vi "数字量输入配置.vi"() -> ()   [LabVIEW 2010]
uses:
  全局量/全局_配置.vi
panel:
  in  "数组":u16[](array[numeric]) format="%x"
  in  "保持输入":bool
  out "同步_A2":i32
  out "同步_A1":i32
  in  "数组_输入值":enum16{"0", "1"}[][](array[ring])
  in  "数组_选择?":bool[][](array[boolean])
  in  "btn_置1_5":bool
  in  "btn_置1_4":bool
  in  "btn_置1_3":bool
  in  "btn_置1_2":bool
  in  "btn_全选_5":bool
  in  "btn_全选_4":bool
  in  "btn_全选_3":bool
  in  "btn_全选_2":bool
  in  "btn_置1_1":bool
  in  "btn_全选_1":bool
  in  "CAN端口":u16
  out "light_80":bool
  out "light_79":bool
  out "light_78":bool
  out "light_77":bool
  out "light_76":bool
  out "light_75":bool
  out "light_74":bool
  out "light_73":bool
  out "light_72":bool
  out "light_71":bool
  out "light_70":bool
  out "light_69":bool
  out "light_68":bool
  out "light_67":bool
  out "light_66":bool
  out "light_65":bool
  in  "输入值_73":enum16{"0", "1"}(ring)
  in  "输入值_80":enum16{"0", "1"}(ring)
  in  "输入值_79":enum16{"0", "1"}(ring)
  in  "输入值_78":enum16{"0", "1"}(ring)
  in  "输入值_77":enum16{"0", "1"}(ring)
  in  "输入值_76":enum16{"0", "1"}(ring)
  in  "输入值_75":enum16{"0", "1"}(ring)
  in  "输入值_74":enum16{"0", "1"}(ring)
  in  "输入值_65":enum16{"0", "1"}(ring)
  in  "输入值_72":enum16{"0", "1"}(ring)
  in  "输入值_71":enum16{"0", "1"}(ring)
  in  "输入值_70":enum16{"0", "1"}(ring)
  in  "输入值_69":enum16{"0", "1"}(ring)
  in  "输入值_68":enum16{"0", "1"}(ring)
  in  "输入值_67":enum16{"0", "1"}(ring)
  in  "输入值_66":enum16{"0", "1"}(ring)
  in  "单选_第73路":bool
  in  "单选_第80路":bool
  in  "单选_第79路":bool
  in  "单选_第78路":bool
  in  "单选_第77路":bool
  in  "单选_第76路":bool
  in  "单选_第75路":bool
  in  "单选_第74路":bool
  in  "单选_第65路":bool
  in  "单选_第72路":bool
  in  "单选_第71路":bool
  in  "单选_第70路":bool
  in  "单选_第69路":bool
  in  "单选_第68路":bool
  in  "单选_第67路":bool
  in  "单选_第66路":bool
  out "light_64":bool
  out "light_63":bool
  out "light_62":bool
  out "light_61":bool
  out "light_60":bool
  out "light_59":bool
  out "light_58":bool
  out "light_57":bool
  out "light_56":bool
  out "light_55":bool
  out "light_54":bool
  out "light_53":bool
  out "light_52":bool
  out "light_51":bool
  out "light_50":bool
  out "light_49":bool
  in  "输入值_57":enum16{"0", "1"}(ring)
  in  "输入值_64":enum16{"0", "1"}(ring)
  in  "输入值_63":enum16{"0", "1"}(ring)
  in  "输入值_62":enum16{"0", "1"}(ring)
  in  "输入值_61":enum16{"0", "1"}(ring)
  in  "输入值_60":enum16{"0", "1"}(ring)
  in  "输入值_59":enum16{"0", "1"}(ring)
  in  "输入值_58":enum16{"0", "1"}(ring)
  in  "输入值_49":enum16{"0", "1"}(ring)
  in  "输入值_56":enum16{"0", "1"}(ring)
  in  "输入值_55":enum16{"0", "1"}(ring)
  in  "输入值_54":enum16{"0", "1"}(ring)
  in  "输入值_53":enum16{"0", "1"}(ring)
  in  "输入值_52":enum16{"0", "1"}(ring)
  in  "输入值_51":enum16{"0", "1"}(ring)
  in  "输入值_50":enum16{"0", "1"}(ring)
  in  "单选_第57路":bool
  in  "单选_第64路":bool
  in  "单选_第63路":bool
  in  "单选_第62路":bool
  in  "单选_第61路":bool
  in  "单选_第60路":bool
  in  "单选_第59路":bool
  in  "单选_第58路":bool
  in  "单选_第49路":bool
  in  "单选_第56路":bool
  in  "单选_第55路":bool
  in  "单选_第54路":bool
  in  "单选_第53路":bool
  in  "单选_第52路":bool
  in  "单选_第51路":bool
  in  "单选_第50路":bool
  out "light_48":bool
  out "light_47":bool
  out "light_46":bool
  out "light_45":bool
  out "light_44":bool
  out "light_43":bool
  out "light_42":bool
  out "light_41":bool
  out "light_40":bool
  out "light_39":bool
  out "light_38":bool
  out "light_37":bool
  out "light_36":bool
  out "light_35":bool
  out "light_34":bool
  out "light_33":bool
  in  "输入值_41":enum16{"0", "1"}(ring)
  in  "输入值_48":enum16{"0", "1"}(ring)
  in  "输入值_47":enum16{"0", "1"}(ring)
  in  "输入值_46":enum16{"0", "1"}(ring)
  in  "输入值_45":enum16{"0", "1"}(ring)
  in  "输入值_44":enum16{"0", "1"}(ring)
  in  "输入值_43":enum16{"0", "1"}(ring)
  in  "输入值_42":enum16{"0", "1"}(ring)
  in  "输入值_33":enum16{"0", "1"}(ring)
  in  "输入值_40":enum16{"0", "1"}(ring)
  in  "输入值_39":enum16{"0", "1"}(ring)
  in  "输入值_38":enum16{"0", "1"}(ring)
  in  "输入值_37":enum16{"0", "1"}(ring)
  in  "输入值_36":enum16{"0", "1"}(ring)
  in  "输入值_35":enum16{"0", "1"}(ring)
  in  "输入值_34":enum16{"0", "1"}(ring)
  in  "单选_第41路":bool
  in  "单选_第48路":bool
  in  "单选_第47路":bool
  in  "单选_第46路":bool
  in  "单选_第45路":bool
  in  "单选_第44路":bool
  in  "单选_第43路":bool
  in  "单选_第42路":bool
  in  "单选_第33路":bool
  in  "单选_第40路":bool
  in  "单选_第39路":bool
  in  "单选_第38路":bool
  in  "单选_第37路":bool
  in  "单选_第36路":bool
  in  "单选_第35路":bool
  in  "单选_第34路":bool
  out "light_32":bool
  out "light_31":bool
  out "light_30":bool
  out "light_29":bool
  out "light_28":bool
  out "light_27":bool
  out "light_26":bool
  out "light_25":bool
  out "light_24":bool
  out "light_23":bool
  out "light_22":bool
  out "light_21":bool
  out "light_20":bool
  out "light_19":bool
  out "light_18":bool
  out "light_17":bool
  in  "输入值_25":enum16{"0", "1"}(ring)
  in  "输入值_32":enum16{"0", "1"}(ring)
  in  "输入值_31":enum16{"0", "1"}(ring)
  in  "输入值_30":enum16{"0", "1"}(ring)
  in  "输入值_29":enum16{"0", "1"}(ring)
  in  "输入值_28":enum16{"0", "1"}(ring)
  in  "输入值_27":enum16{"0", "1"}(ring)
  in  "输入值_26":enum16{"0", "1"}(ring)
  in  "输入值_17":enum16{"0", "1"}(ring)
  in  "输入值_24":enum16{"0", "1"}(ring)
  in  "输入值_23":enum16{"0", "1"}(ring)
  in  "输入值_22":enum16{"0", "1"}(ring)
  in  "输入值_21":enum16{"0", "1"}(ring)
  in  "输入值_20":enum16{"0", "1"}(ring)
  in  "输入值_19":enum16{"0", "1"}(ring)
  in  "输入值_18":enum16{"0", "1"}(ring)
  in  "单选_第25路":bool
  in  "单选_第32路":bool
  in  "单选_第31路":bool
  in  "单选_第30路":bool
  in  "单选_第29路":bool
  in  "单选_第28路":bool
  in  "单选_第27路":bool
  in  "单选_第26路":bool
  in  "单选_第17路":bool
  in  "单选_第24路":bool
  in  "单选_第23路":bool
  in  "单选_第22路":bool
  in  "单选_第21路":bool
  in  "单选_第20路":bool
  in  "单选_第19路":bool
  in  "单选_第18路":bool
  in  "D_IN_5":string[][](table) caption="表格"
  in  "D_IN_4":string[][](table) caption="表格"
  in  "D_IN_3":string[][](table) caption="表格"
  in  "D_IN_2":string[][](table) caption="表格"
  out "light_16":bool
  out "light_15":bool
  out "light_14":bool
  out "light_13":bool
  out "light_12":bool
  out "light_11":bool
  out "light_10":bool
  out "light_9":bool
  out "light_8":bool
  out "light_7":bool
  out "light_6":bool
  out "light_5":bool
  out "light_4":bool
  out "light_3":bool
  out "light_2":bool
  out "light_1":bool
  in  "输入值_9":enum16{"0", "1"}(ring)
  in  "输入值_16":enum16{"0", "1"}(ring)
  in  "输入值_15":enum16{"0", "1"}(ring)
  in  "输入值_14":enum16{"0", "1"}(ring)
  in  "输入值_13":enum16{"0", "1"}(ring)
  in  "输入值_12":enum16{"0", "1"}(ring)
  in  "输入值_11":enum16{"0", "1"}(ring)
  in  "输入值_10":enum16{"0", "1"}(ring)
  in  "输入值_1":enum16{"0", "1"}(ring)
  in  "输入值_8":enum16{"0", "1"}(ring)
  in  "输入值_7":enum16{"0", "1"}(ring)
  in  "输入值_6":enum16{"0", "1"}(ring)
  in  "输入值_5":enum16{"0", "1"}(ring)
  in  "输入值_4":enum16{"0", "1"}(ring)
  in  "输入值_3":enum16{"0", "1"}(ring)
  in  "输入值_2":enum16{"0", "1"}(ring)
  in  "单选_第9路":bool
  in  "单选_第16路":bool
  in  "单选_第15路":bool
  in  "单选_第14路":bool
  in  "单选_第13路":bool
  in  "单选_第12路":bool
  in  "单选_第11路":bool
  in  "单选_第10路":bool
  in  "单选_第1路":bool
  in  "单选_第8路":bool
  in  "单选_第7路":bool
  in  "单选_第6路":bool
  in  "单选_第5路":bool
  in  "单选_第4路":bool
  in  "单选_第3路":bool
  in  "单选_第2路":bool
  in  "D_IN_1":string[][](table) caption="表格"
  out "关闭？":bool
  out "测试结论":string
  in  "btn_置0":bool
  in  "btn_置1":bool
  in  "btn_反选":bool
  in  "btn_全选":bool
  in  "btn_关闭":bool
  in  "btn_开始试验":bool
  # "第一组数字量输入"
  # "第二组数字量输入"
  # "第三组数字量输入"
  # "第四组数字量输入"
  # "第五组数字量输入(I/O)"
  # "测试结论："
  # "5X16"
  # "5X16"
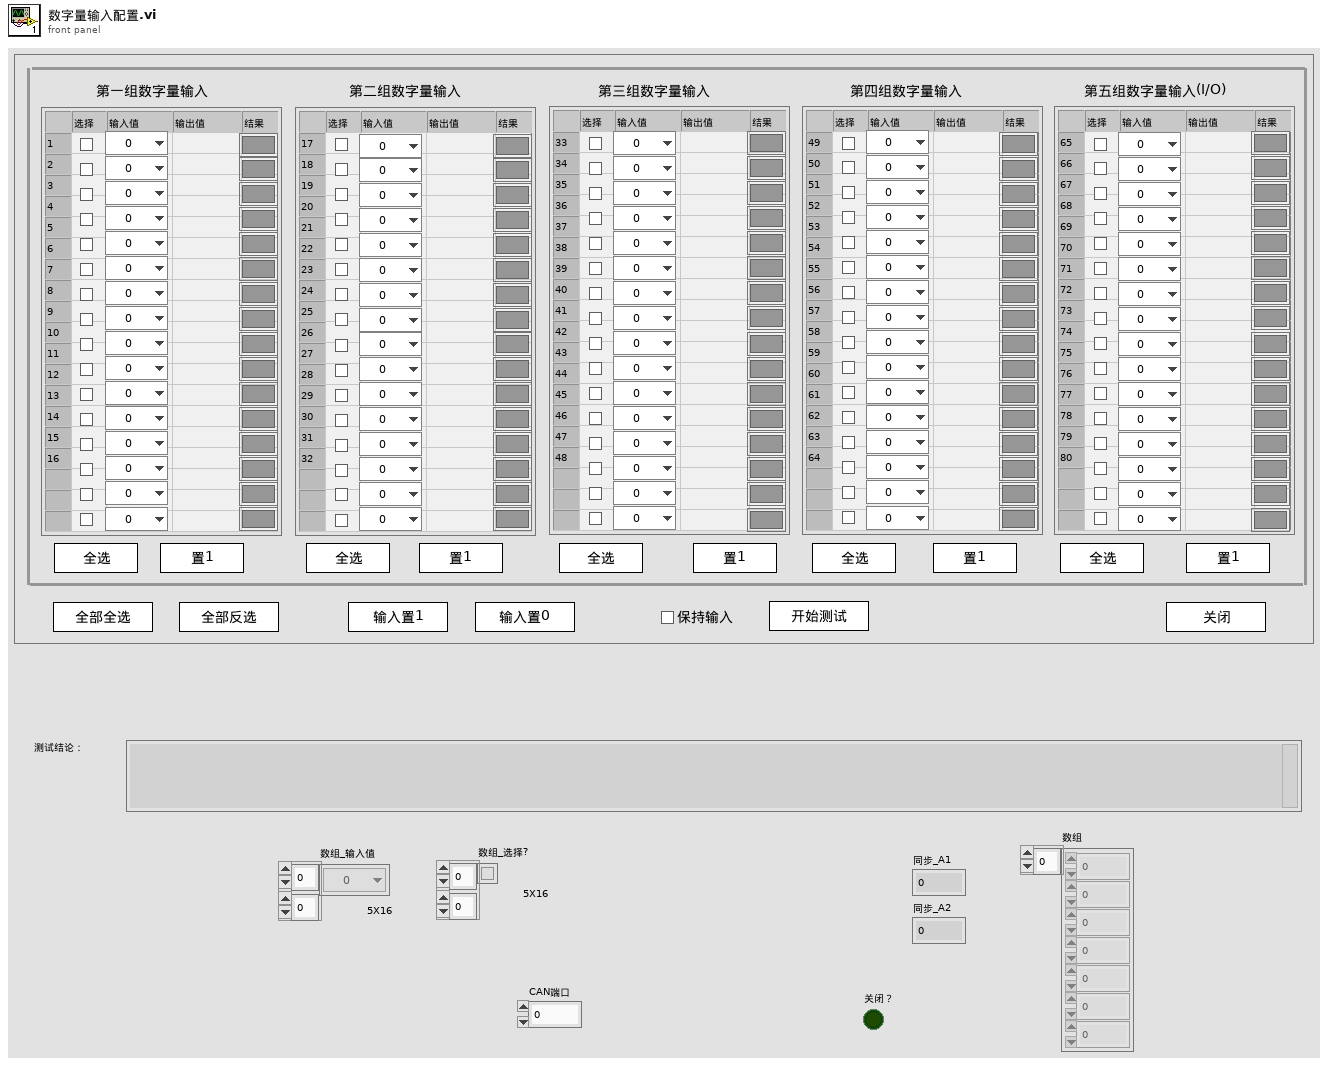
[diagram p1: front panel]
types:
  T1 = enum8{"Enabled", "Disabled", "Disabled and Grayed Out"}
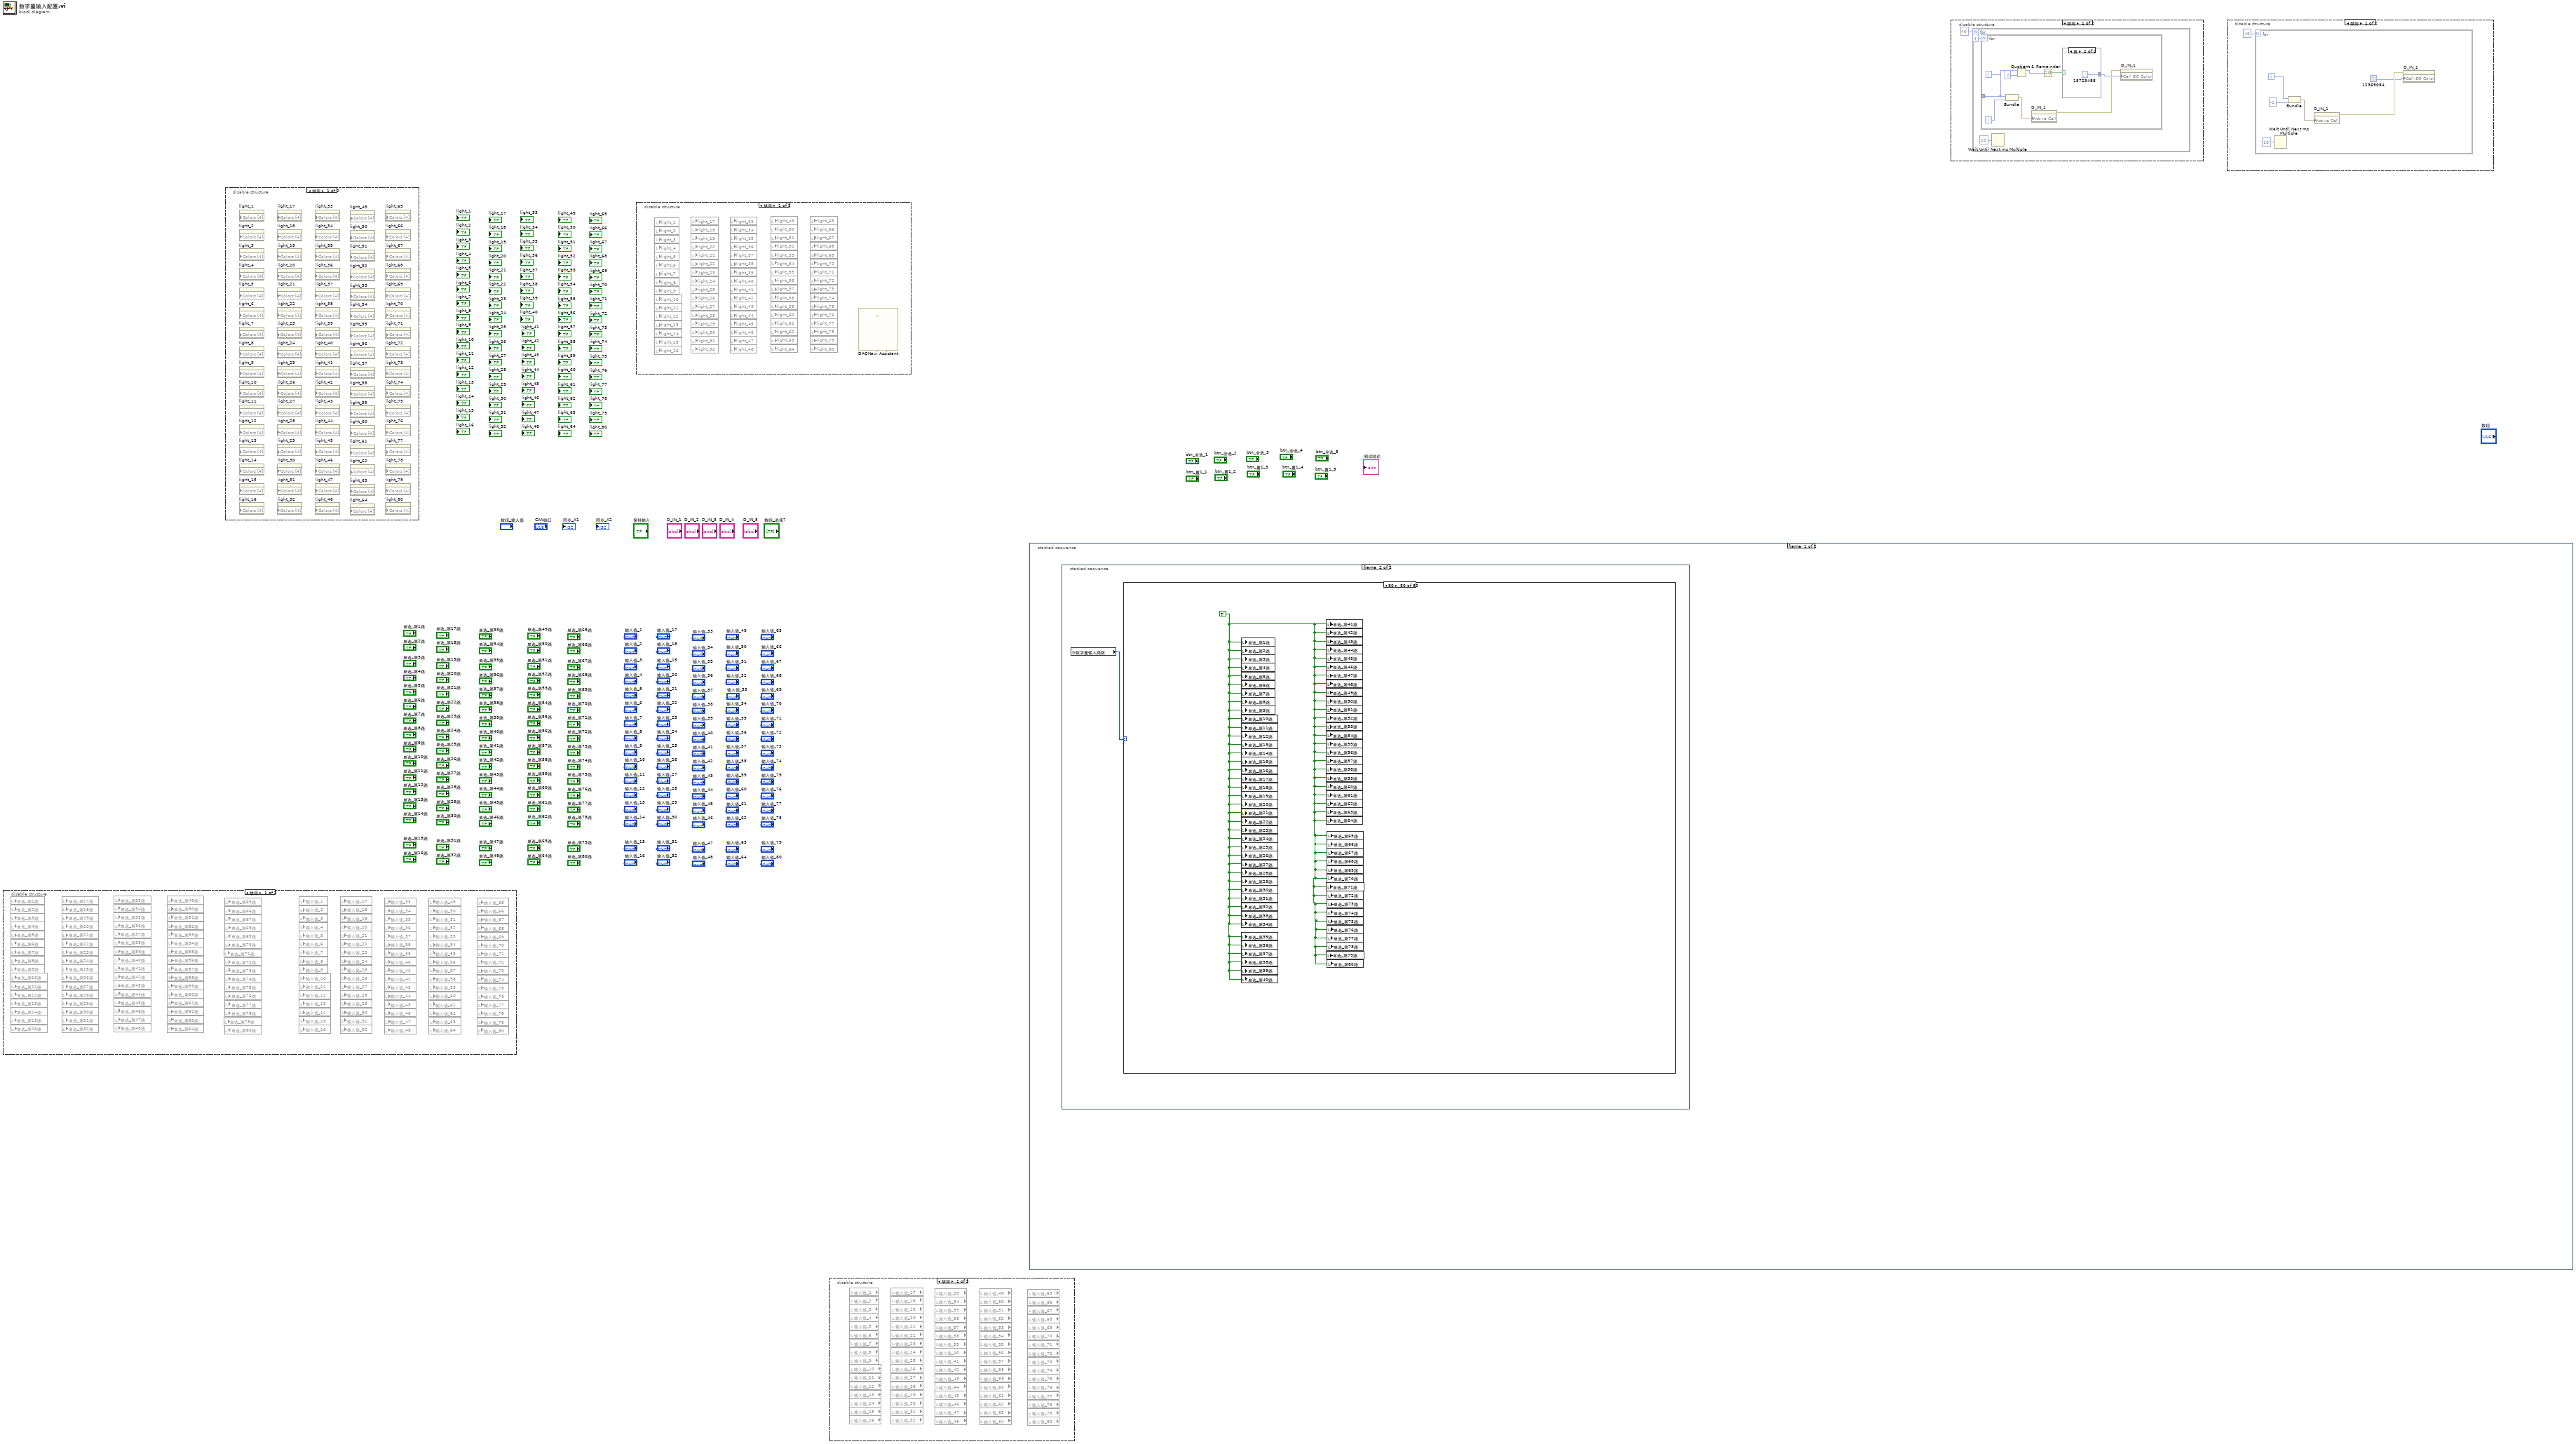
[diagram p0: block diagram]
diagram:
  n1 = disable-structure shown="禁用" {
    frame Disabled {
      n2 = local read "单选_第1路"() -> ()  [unwired: 1 in]
      n3 = local read "单选_第2路"() -> ()  [unwired: 1 in]
      n4 = local read "单选_第3路"() -> ()  [unwired: 1 in]
      n5 = local read "单选_第4路"() -> ()  [unwired: 1 in]
      n6 = local read "单选_第5路"() -> ()  [unwired: 1 in]
      n7 = local read "单选_第6路"() -> ()  [unwired: 1 in]
      n8 = local read "单选_第7路"() -> ()  [unwired: 1 in]
      n9 = local read "单选_第8路"() -> ()  [unwired: 1 in]
      n10 = local read "单选_第9路"() -> ()  [unwired: 1 in]
      n11 = local read "单选_第10路"() -> ()  [unwired: 1 in]
      n12 = local read "单选_第11路"() -> ()  [unwired: 1 in]
      n13 = local read "单选_第12路"() -> ()  [unwired: 1 in]
      n14 = local read "单选_第13路"() -> ()  [unwired: 1 in]
      n15 = local read "单选_第14路"() -> ()  [unwired: 1 in]
      n16 = local read "单选_第15路"() -> ()  [unwired: 1 in]
      n17 = local read "单选_第16路"() -> ()  [unwired: 1 in]
      n18 = local read "单选_第17路"() -> ()  [unwired: 1 in]
      n19 = local read "单选_第18路"() -> ()  [unwired: 1 in]
      n20 = local read "单选_第19路"() -> ()  [unwired: 1 in]
      n21 = local read "单选_第20路"() -> ()  [unwired: 1 in]
      n22 = local read "单选_第21路"() -> ()  [unwired: 1 in]
      n23 = local read "单选_第22路"() -> ()  [unwired: 1 in]
      n24 = local read "单选_第23路"() -> ()  [unwired: 1 in]
      n25 = local read "单选_第24路"() -> ()  [unwired: 1 in]
      n26 = local read "单选_第25路"() -> ()  [unwired: 1 in]
      n27 = local read "单选_第26路"() -> ()  [unwired: 1 in]
      n28 = local read "单选_第27路"() -> ()  [unwired: 1 in]
      n29 = local read "单选_第28路"() -> ()  [unwired: 1 in]
      n30 = local read "单选_第29路"() -> ()  [unwired: 1 in]
      n31 = local read "单选_第30路"() -> ()  [unwired: 1 in]
      n32 = local read "单选_第31路"() -> ()  [unwired: 1 in]
      n33 = local read "单选_第32路"() -> ()  [unwired: 1 in]
      n34 = local read "单选_第33路"() -> ()  [unwired: 1 in]
      n35 = local read "单选_第34路"() -> ()  [unwired: 1 in]
      n36 = local read "单选_第35路"() -> ()  [unwired: 1 in]
      n37 = local read "单选_第36路"() -> ()  [unwired: 1 in]
      n38 = local read "单选_第37路"() -> ()  [unwired: 1 in]
      n39 = local read "单选_第38路"() -> ()  [unwired: 1 in]
      n40 = local read "单选_第39路"() -> ()  [unwired: 1 in]
      n41 = local read "单选_第40路"() -> ()  [unwired: 1 in]
      n42 = local read "单选_第41路"() -> ()  [unwired: 1 in]
      n43 = local read "单选_第42路"() -> ()  [unwired: 1 in]
      n44 = local read "单选_第43路"() -> ()  [unwired: 1 in]
      n45 = local read "单选_第44路"() -> ()  [unwired: 1 in]
      n46 = local read "单选_第45路"() -> ()  [unwired: 1 in]
      n47 = local read "单选_第46路"() -> ()  [unwired: 1 in]
      n48 = local read "单选_第47路"() -> ()  [unwired: 1 in]
      n49 = local read "单选_第48路"() -> ()  [unwired: 1 in]
      n50 = local read "单选_第49路"() -> ()  [unwired: 1 in]
      n51 = local read "单选_第50路"() -> ()  [unwired: 1 in]
      n52 = local read "单选_第51路"() -> ()  [unwired: 1 in]
      n53 = local read "单选_第52路"() -> ()  [unwired: 1 in]
      n54 = local read "单选_第53路"() -> ()  [unwired: 1 in]
      n55 = local read "单选_第54路"() -> ()  [unwired: 1 in]
      n56 = local read "单选_第55路"() -> ()  [unwired: 1 in]
      n57 = local read "单选_第56路"() -> ()  [unwired: 1 in]
      n58 = local read "单选_第57路"() -> ()  [unwired: 1 in]
      n59 = local read "单选_第58路"() -> ()  [unwired: 1 in]
      n60 = local read "单选_第59路"() -> ()  [unwired: 1 in]
      n61 = local read "单选_第60路"() -> ()  [unwired: 1 in]
      n62 = local read "单选_第61路"() -> ()  [unwired: 1 in]
      n63 = local read "单选_第62路"() -> ()  [unwired: 1 in]
      n64 = local read "单选_第63路"() -> ()  [unwired: 1 in]
      n65 = local read "单选_第64路"() -> ()  [unwired: 1 in]
      n66 = local read "单选_第71路"() -> ()  [unwired: 1 in]
      n67 = local read "单选_第79路"() -> ()  [unwired: 1 in]
      n68 = local read "单选_第65路"() -> ()  [unwired: 1 in]
      n69 = local read "单选_第66路"() -> ()  [unwired: 1 in]
      n70 = local read "单选_第67路"() -> ()  [unwired: 1 in]
      n71 = local read "单选_第68路"() -> ()  [unwired: 1 in]
      n72 = local read "单选_第69路"() -> ()  [unwired: 1 in]
      n73 = local read "单选_第70路"() -> ()  [unwired: 1 in]
      n74 = local read "单选_第72路"() -> ()  [unwired: 1 in]
      n75 = local read "单选_第73路"() -> ()  [unwired: 1 in]
      n76 = local read "单选_第74路"() -> ()  [unwired: 1 in]
      n77 = local read "单选_第75路"() -> ()  [unwired: 1 in]
      n78 = local read "单选_第76路"() -> ()  [unwired: 1 in]
      n79 = local read "单选_第77路"() -> ()  [unwired: 1 in]
      n80 = local read "单选_第78路"() -> ()  [unwired: 1 in]
      n81 = local read "单选_第80路"() -> ()  [unwired: 1 in]
      n82 = local read "输入值_1"() -> ()  [unwired: 1 in]
      n83 = local read "输入值_2"() -> ()  [unwired: 1 in]
      n84 = local read "输入值_3"() -> ()  [unwired: 1 in]
      n85 = local read "输入值_4"() -> ()  [unwired: 1 in]
      n86 = local read "输入值_5"() -> ()  [unwired: 1 in]
      n87 = local read "输入值_6"() -> ()  [unwired: 1 in]
      n88 = local read "输入值_7"() -> ()  [unwired: 1 in]
      n89 = local read "输入值_8"() -> ()  [unwired: 1 in]
      n90 = local read "输入值_9"() -> ()  [unwired: 1 in]
      n91 = local read "输入值_10"() -> ()  [unwired: 1 in]
      n92 = local read "输入值_11"() -> ()  [unwired: 1 in]
      n93 = local read "输入值_12"() -> ()  [unwired: 1 in]
      n94 = local read "输入值_13"() -> ()  [unwired: 1 in]
      n95 = local read "输入值_14"() -> ()  [unwired: 1 in]
      n96 = local read "输入值_15"() -> ()  [unwired: 1 in]
      n97 = local read "输入值_16"() -> ()  [unwired: 1 in]
      n98 = local read "输入值_17"() -> ()  [unwired: 1 in]
      n99 = local read "输入值_18"() -> ()  [unwired: 1 in]
      n100 = local read "输入值_19"() -> ()  [unwired: 1 in]
      n101 = local read "输入值_20"() -> ()  [unwired: 1 in]
      n102 = local read "输入值_21"() -> ()  [unwired: 1 in]
      n103 = local read "输入值_22"() -> ()  [unwired: 1 in]
      n104 = local read "输入值_23"() -> ()  [unwired: 1 in]
      n105 = local read "输入值_24"() -> ()  [unwired: 1 in]
      n106 = local read "输入值_25"() -> ()  [unwired: 1 in]
      n107 = local read "输入值_26"() -> ()  [unwired: 1 in]
      n108 = local read "输入值_27"() -> ()  [unwired: 1 in]
      n109 = local read "输入值_28"() -> ()  [unwired: 1 in]
      n110 = local read "输入值_29"() -> ()  [unwired: 1 in]
      n111 = local read "输入值_30"() -> ()  [unwired: 1 in]
      n112 = local read "输入值_31"() -> ()  [unwired: 1 in]
      n113 = local read "输入值_32"() -> ()  [unwired: 1 in]
      n114 = local read "输入值_33"() -> ()  [unwired: 1 in]
      n115 = local read "输入值_34"() -> ()  [unwired: 1 in]
      n116 = local read "输入值_35"() -> ()  [unwired: 1 in]
      n117 = local read "输入值_36"() -> ()  [unwired: 1 in]
      n118 = local read "输入值_37"() -> ()  [unwired: 1 in]
      n119 = local read "输入值_38"() -> ()  [unwired: 1 in]
      n120 = local read "输入值_39"() -> ()  [unwired: 1 in]
      n121 = local read "输入值_40"() -> ()  [unwired: 1 in]
      n122 = local read "输入值_41"() -> ()  [unwired: 1 in]
      n123 = local read "输入值_42"() -> ()  [unwired: 1 in]
      n124 = local read "输入值_43"() -> ()  [unwired: 1 in]
      n125 = local read "输入值_44"() -> ()  [unwired: 1 in]
      n126 = local read "输入值_45"() -> ()  [unwired: 1 in]
      n127 = local read "输入值_46"() -> ()  [unwired: 1 in]
      n128 = local read "输入值_47"() -> ()  [unwired: 1 in]
      n129 = local read "输入值_48"() -> ()  [unwired: 1 in]
      n130 = local read "输入值_49"() -> ()  [unwired: 1 in]
      n131 = local read "输入值_50"() -> ()  [unwired: 1 in]
      n132 = local read "输入值_51"() -> ()  [unwired: 1 in]
      n133 = local read "输入值_52"() -> ()  [unwired: 1 in]
      n134 = local read "输入值_53"() -> ()  [unwired: 1 in]
      n135 = local read "输入值_54"() -> ()  [unwired: 1 in]
      n136 = local read "输入值_55"() -> ()  [unwired: 1 in]
      n137 = local read "输入值_56"() -> ()  [unwired: 1 in]
      n138 = local read "输入值_57"() -> ()  [unwired: 1 in]
      n139 = local read "输入值_58"() -> ()  [unwired: 1 in]
      n140 = local read "输入值_59"() -> ()  [unwired: 1 in]
      n141 = local read "输入值_60"() -> ()  [unwired: 1 in]
      n142 = local read "输入值_61"() -> ()  [unwired: 1 in]
      n143 = local read "输入值_62"() -> ()  [unwired: 1 in]
      n144 = local read "输入值_63"() -> ()  [unwired: 1 in]
      n145 = local read "输入值_64"() -> ()  [unwired: 1 in]
      n146 = local read "输入值_65"() -> ()  [unwired: 1 in]
      n147 = local read "输入值_66"() -> ()  [unwired: 1 in]
      n148 = local read "输入值_67"() -> ()  [unwired: 1 in]
      n149 = local read "输入值_68"() -> ()  [unwired: 1 in]
      n150 = local read "输入值_69"() -> ()  [unwired: 1 in]
      n151 = local read "输入值_70"() -> ()  [unwired: 1 in]
      n152 = local read "输入值_71"() -> ()  [unwired: 1 in]
      n153 = local read "输入值_72"() -> ()  [unwired: 1 in]
      n154 = local read "输入值_73"() -> ()  [unwired: 1 in]
      n155 = local read "输入值_74"() -> ()  [unwired: 1 in]
      n156 = local read "输入值_75"() -> ()  [unwired: 1 in]
      n157 = local read "输入值_76"() -> ()  [unwired: 1 in]
      n158 = local read "输入值_77"() -> ()  [unwired: 1 in]
      n159 = local read "输入值_78"() -> ()  [unwired: 1 in]
      n160 = local read "输入值_79"() -> ()  [unwired: 1 in]
      n161 = local read "输入值_80"() -> ()  [unwired: 1 in]
    }
    frame Enabled {
    }
  }
  n162 = disable-structure shown="禁用" {
    frame Disabled {
      n163 = property on="light_1" class="Bool (严格)" props=["Colors [4]"]() -> ()  [unwired: 3 in, 2 out]
      n164 = property on="light_2" class="Bool (严格)" props=["Colors [4]"]() -> ()  [unwired: 3 in, 2 out]
      n165 = property on="light_3" class="Bool (严格)" props=["Colors [4]"]() -> ()  [unwired: 3 in, 2 out]
      n166 = property on="light_4" class="Bool (严格)" props=["Colors [4]"]() -> ()  [unwired: 3 in, 2 out]
      n167 = property on="light_5" class="Bool (严格)" props=["Colors [4]"]() -> ()  [unwired: 3 in, 2 out]
      n168 = property on="light_6" class="Bool (严格)" props=["Colors [4]"]() -> ()  [unwired: 3 in, 2 out]
      n169 = property on="light_7" class="Bool (严格)" props=["Colors [4]"]() -> ()  [unwired: 3 in, 2 out]
      n170 = property on="light_8" class="Bool (严格)" props=["Colors [4]"]() -> ()  [unwired: 3 in, 2 out]
      n171 = property on="light_9" class="Bool (严格)" props=["Colors [4]"]() -> ()  [unwired: 3 in, 2 out]
      n172 = property on="light_10" class="Bool (严格)" props=["Colors [4]"]() -> ()  [unwired: 3 in, 2 out]
      n173 = property on="light_11" class="Bool (严格)" props=["Colors [4]"]() -> ()  [unwired: 3 in, 2 out]
      n174 = property on="light_12" class="Bool (严格)" props=["Colors [4]"]() -> ()  [unwired: 3 in, 2 out]
      n175 = property on="light_13" class="Bool (严格)" props=["Colors [4]"]() -> ()  [unwired: 3 in, 2 out]
      n176 = property on="light_14" class="Bool (严格)" props=["Colors [4]"]() -> ()  [unwired: 3 in, 2 out]
      n177 = property on="light_15" class="Bool (严格)" props=["Colors [4]"]() -> ()  [unwired: 3 in, 2 out]
      n178 = property on="light_16" class="Bool (严格)" props=["Colors [4]"]() -> ()  [unwired: 3 in, 2 out]
      n179 = property on="light_17" class="Bool (严格)" props=["Colors [4]"]() -> ()  [unwired: 3 in, 2 out]
      n180 = property on="light_18" class="Bool (严格)" props=["Colors [4]"]() -> ()  [unwired: 3 in, 2 out]
      n181 = property on="light_19" class="Bool (严格)" props=["Colors [4]"]() -> ()  [unwired: 3 in, 2 out]
      n182 = property on="light_20" class="Bool (严格)" props=["Colors [4]"]() -> ()  [unwired: 3 in, 2 out]
      n183 = property on="light_21" class="Bool (严格)" props=["Colors [4]"]() -> ()  [unwired: 3 in, 2 out]
      n184 = property on="light_22" class="Bool (严格)" props=["Colors [4]"]() -> ()  [unwired: 3 in, 2 out]
      n185 = property on="light_23" class="Bool (严格)" props=["Colors [4]"]() -> ()  [unwired: 3 in, 2 out]
      n186 = property on="light_24" class="Bool (严格)" props=["Colors [4]"]() -> ()  [unwired: 3 in, 2 out]
      n187 = property on="light_25" class="Bool (严格)" props=["Colors [4]"]() -> ()  [unwired: 3 in, 2 out]
      n188 = property on="light_26" class="Bool (严格)" props=["Colors [4]"]() -> ()  [unwired: 3 in, 2 out]
      n189 = property on="light_27" class="Bool (严格)" props=["Colors [4]"]() -> ()  [unwired: 3 in, 2 out]
      n190 = property on="light_28" class="Bool (严格)" props=["Colors [4]"]() -> ()  [unwired: 3 in, 2 out]
      n191 = property on="light_29" class="Bool (严格)" props=["Colors [4]"]() -> ()  [unwired: 3 in, 2 out]
      n192 = property on="light_30" class="Bool (严格)" props=["Colors [4]"]() -> ()  [unwired: 3 in, 2 out]
      n193 = property on="light_31" class="Bool (严格)" props=["Colors [4]"]() -> ()  [unwired: 3 in, 2 out]
      n194 = property on="light_32" class="Bool (严格)" props=["Colors [4]"]() -> ()  [unwired: 3 in, 2 out]
      n195 = property on="light_33" class="Bool (严格)" props=["Colors [4]"]() -> ()  [unwired: 3 in, 2 out]
      n196 = property on="light_34" class="Bool (严格)" props=["Colors [4]"]() -> ()  [unwired: 3 in, 2 out]
      n197 = property on="light_35" class="Bool (严格)" props=["Colors [4]"]() -> ()  [unwired: 3 in, 2 out]
      n198 = property on="light_36" class="Bool (严格)" props=["Colors [4]"]() -> ()  [unwired: 3 in, 2 out]
      n199 = property on="light_37" class="Bool (严格)" props=["Colors [4]"]() -> ()  [unwired: 3 in, 2 out]
      n200 = property on="light_38" class="Bool (严格)" props=["Colors [4]"]() -> ()  [unwired: 3 in, 2 out]
      n201 = property on="light_39" class="Bool (严格)" props=["Colors [4]"]() -> ()  [unwired: 3 in, 2 out]
      n202 = property on="light_40" class="Bool (严格)" props=["Colors [4]"]() -> ()  [unwired: 3 in, 2 out]
      n203 = property on="light_41" class="Bool (严格)" props=["Colors [4]"]() -> ()  [unwired: 3 in, 2 out]
      n204 = property on="light_42" class="Bool (严格)" props=["Colors [4]"]() -> ()  [unwired: 3 in, 2 out]
      n205 = property on="light_43" class="Bool (严格)" props=["Colors [4]"]() -> ()  [unwired: 3 in, 2 out]
      n206 = property on="light_44" class="Bool (严格)" props=["Colors [4]"]() -> ()  [unwired: 3 in, 2 out]
      n207 = property on="light_45" class="Bool (严格)" props=["Colors [4]"]() -> ()  [unwired: 3 in, 2 out]
      n208 = property on="light_46" class="Bool (严格)" props=["Colors [4]"]() -> ()  [unwired: 3 in, 2 out]
      n209 = property on="light_47" class="Bool (严格)" props=["Colors [4]"]() -> ()  [unwired: 3 in, 2 out]
      n210 = property on="light_48" class="Bool (严格)" props=["Colors [4]"]() -> ()  [unwired: 3 in, 2 out]
      n211 = property on="light_49" class="Bool (严格)" props=["Colors [4]"]() -> ()  [unwired: 3 in, 2 out]
      n212 = property on="light_50" class="Bool (严格)" props=["Colors [4]"]() -> ()  [unwired: 3 in, 2 out]
      n213 = property on="light_51" class="Bool (严格)" props=["Colors [4]"]() -> ()  [unwired: 3 in, 2 out]
      n214 = property on="light_52" class="Bool (严格)" props=["Colors [4]"]() -> ()  [unwired: 3 in, 2 out]
      n215 = property on="light_53" class="Bool (严格)" props=["Colors [4]"]() -> ()  [unwired: 3 in, 2 out]
      n216 = property on="light_54" class="Bool (严格)" props=["Colors [4]"]() -> ()  [unwired: 3 in, 2 out]
      n217 = property on="light_55" class="Bool (严格)" props=["Colors [4]"]() -> ()  [unwired: 3 in, 2 out]
      n218 = property on="light_56" class="Bool (严格)" props=["Colors [4]"]() -> ()  [unwired: 3 in, 2 out]
      n219 = property on="light_57" class="Bool (严格)" props=["Colors [4]"]() -> ()  [unwired: 3 in, 2 out]
      n220 = property on="light_58" class="Bool (严格)" props=["Colors [4]"]() -> ()  [unwired: 3 in, 2 out]
      n221 = property on="light_59" class="Bool (严格)" props=["Colors [4]"]() -> ()  [unwired: 3 in, 2 out]
      n222 = property on="light_60" class="Bool (严格)" props=["Colors [4]"]() -> ()  [unwired: 3 in, 2 out]
      n223 = property on="light_61" class="Bool (严格)" props=["Colors [4]"]() -> ()  [unwired: 3 in, 2 out]
      n224 = property on="light_62" class="Bool (严格)" props=["Colors [4]"]() -> ()  [unwired: 3 in, 2 out]
      n225 = property on="light_63" class="Bool (严格)" props=["Colors [4]"]() -> ()  [unwired: 3 in, 2 out]
      n226 = property on="light_64" class="Bool (严格)" props=["Colors [4]"]() -> ()  [unwired: 3 in, 2 out]
      n227 = property on="light_65" class="Bool (严格)" props=["Colors [4]"]() -> ()  [unwired: 3 in, 2 out]
      n228 = property on="light_66" class="Bool (严格)" props=["Colors [4]"]() -> ()  [unwired: 3 in, 2 out]
      n229 = property on="light_67" class="Bool (严格)" props=["Colors [4]"]() -> ()  [unwired: 3 in, 2 out]
      n230 = property on="light_68" class="Bool (严格)" props=["Colors [4]"]() -> ()  [unwired: 3 in, 2 out]
      n231 = property on="light_69" class="Bool (严格)" props=["Colors [4]"]() -> ()  [unwired: 3 in, 2 out]
      n232 = property on="light_70" class="Bool (严格)" props=["Colors [4]"]() -> ()  [unwired: 3 in, 2 out]
      n233 = property on="light_71" class="Bool (严格)" props=["Colors [4]"]() -> ()  [unwired: 3 in, 2 out]
      n234 = property on="light_72" class="Bool (严格)" props=["Colors [4]"]() -> ()  [unwired: 3 in, 2 out]
      n235 = property on="light_73" class="Bool (严格)" props=["Colors [4]"]() -> ()  [unwired: 3 in, 2 out]
      n236 = property on="light_74" class="Bool (严格)" props=["Colors [4]"]() -> ()  [unwired: 3 in, 2 out]
      n237 = property on="light_75" class="Bool (严格)" props=["Colors [4]"]() -> ()  [unwired: 3 in, 2 out]
      n238 = property on="light_76" class="Bool (严格)" props=["Colors [4]"]() -> ()  [unwired: 3 in, 2 out]
      n239 = property on="light_77" class="Bool (严格)" props=["Colors [4]"]() -> ()  [unwired: 3 in, 2 out]
      n240 = property on="light_78" class="Bool (严格)" props=["Colors [4]"]() -> ()  [unwired: 3 in, 2 out]
      n241 = property on="light_79" class="Bool (严格)" props=["Colors [4]"]() -> ()  [unwired: 3 in, 2 out]
      n242 = property on="light_80" class="Bool (严格)" props=["Colors [4]"]() -> ()  [unwired: 3 in, 2 out]
    }
    frame Enabled {
    }
  }
  n243 = disable-structure shown="禁用" {
    frame Disabled {
      n244 = local read "light_1"() -> ()  [unwired: 1 in]
      n245 = local read "light_2"() -> ()  [unwired: 1 in]
      n246 = local read "light_3"() -> ()  [unwired: 1 in]
      n247 = local read "light_4"() -> ()  [unwired: 1 in]
      n248 = local read "light_5"() -> ()  [unwired: 1 in]
      n249 = local read "light_6"() -> ()  [unwired: 1 in]
      n250 = local read "light_7"() -> ()  [unwired: 1 in]
      n251 = local read "light_8"() -> ()  [unwired: 1 in]
      n252 = local read "light_9"() -> ()  [unwired: 1 in]
      n253 = local read "light_10"() -> ()  [unwired: 1 in]
      n254 = local read "light_11"() -> ()  [unwired: 1 in]
      n255 = local read "light_12"() -> ()  [unwired: 1 in]
      n256 = local read "light_13"() -> ()  [unwired: 1 in]
      n257 = local read "light_14"() -> ()  [unwired: 1 in]
      n258 = local read "light_15"() -> ()  [unwired: 1 in]
      n259 = local read "light_16"() -> ()  [unwired: 1 in]
      n260 = local read "light_17"() -> ()  [unwired: 1 in]
      n261 = local read "light_18"() -> ()  [unwired: 1 in]
      n262 = local read "light_19"() -> ()  [unwired: 1 in]
      n263 = local read "light_20"() -> ()  [unwired: 1 in]
      n264 = local read "light_21"() -> ()  [unwired: 1 in]
      n265 = local read "light_22"() -> ()  [unwired: 1 in]
      n266 = local read "light_23"() -> ()  [unwired: 1 in]
      n267 = local read "light_24"() -> ()  [unwired: 1 in]
      n268 = local read "light_25"() -> ()  [unwired: 1 in]
      n269 = local read "light_26"() -> ()  [unwired: 1 in]
      n270 = local read "light_27"() -> ()  [unwired: 1 in]
      n271 = local read "light_28"() -> ()  [unwired: 1 in]
      n272 = local read "light_29"() -> ()  [unwired: 1 in]
      n273 = local read "light_30"() -> ()  [unwired: 1 in]
      n274 = local read "light_31"() -> ()  [unwired: 1 in]
      n275 = local read "light_32"() -> ()  [unwired: 1 in]
      n276 = local read "light_33"() -> ()  [unwired: 1 in]
      n277 = local read "light_34"() -> ()  [unwired: 1 in]
      n278 = local read "light_35"() -> ()  [unwired: 1 in]
      n279 = local read "light_36"() -> ()  [unwired: 1 in]
      n280 = local read "light_37"() -> ()  [unwired: 1 in]
      n281 = local read "light_38"() -> ()  [unwired: 1 in]
      n282 = local read "light_39"() -> ()  [unwired: 1 in]
      n283 = local read "light_40"() -> ()  [unwired: 1 in]
      n284 = local read "light_41"() -> ()  [unwired: 1 in]
      n285 = local read "light_42"() -> ()  [unwired: 1 in]
      n286 = local read "light_43"() -> ()  [unwired: 1 in]
      n287 = local read "light_44"() -> ()  [unwired: 1 in]
      n288 = local read "light_45"() -> ()  [unwired: 1 in]
      n289 = local read "light_46"() -> ()  [unwired: 1 in]
      n290 = local read "light_47"() -> ()  [unwired: 1 in]
      n291 = local read "light_48"() -> ()  [unwired: 1 in]
      n292 = local read "light_49"() -> ()  [unwired: 1 in]
      n293 = local read "light_50"() -> ()  [unwired: 1 in]
      n294 = local read "light_51"() -> ()  [unwired: 1 in]
      n295 = local read "light_52"() -> ()  [unwired: 1 in]
      n296 = local read "light_53"() -> ()  [unwired: 1 in]
      n297 = local read "light_54"() -> ()  [unwired: 1 in]
      n298 = local read "light_55"() -> ()  [unwired: 1 in]
      n299 = local read "light_56"() -> ()  [unwired: 1 in]
      n300 = local read "light_57"() -> ()  [unwired: 1 in]
      n301 = local read "light_58"() -> ()  [unwired: 1 in]
      n302 = local read "light_59"() -> ()  [unwired: 1 in]
      n303 = local read "light_60"() -> ()  [unwired: 1 in]
      n304 = local read "light_61"() -> ()  [unwired: 1 in]
      n305 = local read "light_62"() -> ()  [unwired: 1 in]
      n306 = local read "light_63"() -> ()  [unwired: 1 in]
      n307 = local read "light_64"() -> ()  [unwired: 1 in]
      n308 = local read "light_65"() -> ()  [unwired: 1 in]
      n309 = local read "light_66"() -> ()  [unwired: 1 in]
      n310 = local read "light_67"() -> ()  [unwired: 1 in]
      n311 = local read "light_68"() -> ()  [unwired: 1 in]
      n312 = local read "light_69"() -> ()  [unwired: 1 in]
      n313 = local read "light_70"() -> ()  [unwired: 1 in]
      n314 = local read "light_71"() -> ()  [unwired: 1 in]
      n315 = local read "light_72"() -> ()  [unwired: 1 in]
      n316 = local read "light_73"() -> ()  [unwired: 1 in]
      n317 = local read "light_74"() -> ()  [unwired: 1 in]
      n318 = local read "light_75"() -> ()  [unwired: 1 in]
      n319 = local read "light_76"() -> ()  [unwired: 1 in]
      n320 = local read "light_77"() -> ()  [unwired: 1 in]
      n321 = local read "light_78"() -> ()  [unwired: 1 in]
      n322 = local read "light_79"() -> ()  [unwired: 1 in]
      n323 = local read "light_80"() -> ()  [unwired: 1 in]
      n324 = call "DAQNavi Assistant"() -> ()  [unwired: 2 in, 18 out]
    }
    frame Enabled {
    }
  }
  n325 = disable-structure shown="禁用" {
    frame Disabled {
      n326 = local read "输入值_1"() -> ()  [unwired: 1 out]
      n327 = local read "输入值_2"() -> ()  [unwired: 1 out]
      n328 = local read "输入值_3"() -> ()  [unwired: 1 out]
      n329 = local read "输入值_4"() -> ()  [unwired: 1 out]
      n330 = local read "输入值_5"() -> ()  [unwired: 1 out]
      n331 = local read "输入值_6"() -> ()  [unwired: 1 out]
      n332 = local read "输入值_7"() -> ()  [unwired: 1 out]
      n333 = local read "输入值_8"() -> ()  [unwired: 1 out]
      n334 = local read "输入值_9"() -> ()  [unwired: 1 out]
      n335 = local read "输入值_10"() -> ()  [unwired: 1 out]
      n336 = local read "输入值_11"() -> ()  [unwired: 1 out]
      n337 = local read "输入值_12"() -> ()  [unwired: 1 out]
      n338 = local read "输入值_13"() -> ()  [unwired: 1 out]
      n339 = local read "输入值_14"() -> ()  [unwired: 1 out]
      n340 = local read "输入值_15"() -> ()  [unwired: 1 out]
      n341 = local read "输入值_16"() -> ()  [unwired: 1 out]
      n342 = local read "输入值_17"() -> ()  [unwired: 1 out]
      n343 = local read "输入值_18"() -> ()  [unwired: 1 out]
      n344 = local read "输入值_19"() -> ()  [unwired: 1 out]
      n345 = local read "输入值_20"() -> ()  [unwired: 1 out]
      n346 = local read "输入值_21"() -> ()  [unwired: 1 out]
      n347 = local read "输入值_22"() -> ()  [unwired: 1 out]
      n348 = local read "输入值_23"() -> ()  [unwired: 1 out]
      n349 = local read "输入值_24"() -> ()  [unwired: 1 out]
      n350 = local read "输入值_25"() -> ()  [unwired: 1 out]
      n351 = local read "输入值_26"() -> ()  [unwired: 1 out]
      n352 = local read "输入值_27"() -> ()  [unwired: 1 out]
      n353 = local read "输入值_28"() -> ()  [unwired: 1 out]
      n354 = local read "输入值_29"() -> ()  [unwired: 1 out]
      n355 = local read "输入值_30"() -> ()  [unwired: 1 out]
      n356 = local read "输入值_31"() -> ()  [unwired: 1 out]
      n357 = local read "输入值_32"() -> ()  [unwired: 1 out]
      n358 = local read "输入值_33"() -> ()  [unwired: 1 out]
      n359 = local read "输入值_34"() -> ()  [unwired: 1 out]
      n360 = local read "输入值_35"() -> ()  [unwired: 1 out]
      n361 = local read "输入值_36"() -> ()  [unwired: 1 out]
      n362 = local read "输入值_37"() -> ()  [unwired: 1 out]
      n363 = local read "输入值_38"() -> ()  [unwired: 1 out]
      n364 = local read "输入值_39"() -> ()  [unwired: 1 out]
      n365 = local read "输入值_40"() -> ()  [unwired: 1 out]
      n366 = local read "输入值_41"() -> ()  [unwired: 1 out]
      n367 = local read "输入值_42"() -> ()  [unwired: 1 out]
      n368 = local read "输入值_43"() -> ()  [unwired: 1 out]
      n369 = local read "输入值_44"() -> ()  [unwired: 1 out]
      n370 = local read "输入值_45"() -> ()  [unwired: 1 out]
      n371 = local read "输入值_46"() -> ()  [unwired: 1 out]
      n372 = local read "输入值_47"() -> ()  [unwired: 1 out]
      n373 = local read "输入值_48"() -> ()  [unwired: 1 out]
      n374 = local read "输入值_49"() -> ()  [unwired: 1 out]
      n375 = local read "输入值_50"() -> ()  [unwired: 1 out]
      n376 = local read "输入值_51"() -> ()  [unwired: 1 out]
      n377 = local read "输入值_52"() -> ()  [unwired: 1 out]
      n378 = local read "输入值_53"() -> ()  [unwired: 1 out]
      n379 = local read "输入值_54"() -> ()  [unwired: 1 out]
      n380 = local read "输入值_55"() -> ()  [unwired: 1 out]
      n381 = local read "输入值_56"() -> ()  [unwired: 1 out]
      n382 = local read "输入值_57"() -> ()  [unwired: 1 out]
      n383 = local read "输入值_58"() -> ()  [unwired: 1 out]
      n384 = local read "输入值_59"() -> ()  [unwired: 1 out]
      n385 = local read "输入值_60"() -> ()  [unwired: 1 out]
      n386 = local read "输入值_61"() -> ()  [unwired: 1 out]
      n387 = local read "输入值_62"() -> ()  [unwired: 1 out]
      n388 = local read "输入值_63"() -> ()  [unwired: 1 out]
      n389 = local read "输入值_64"() -> ()  [unwired: 1 out]
      n390 = local read "输入值_65"() -> ()  [unwired: 1 out]
      n391 = local read "输入值_66"() -> ()  [unwired: 1 out]
      n392 = local read "输入值_67"() -> ()  [unwired: 1 out]
      n393 = local read "输入值_68"() -> ()  [unwired: 1 out]
      n394 = local read "输入值_69"() -> ()  [unwired: 1 out]
      n395 = local read "输入值_70"() -> ()  [unwired: 1 out]
      n396 = local read "输入值_71"() -> ()  [unwired: 1 out]
      n397 = local read "输入值_72"() -> ()  [unwired: 1 out]
      n398 = local read "输入值_73"() -> ()  [unwired: 1 out]
      n399 = local read "输入值_74"() -> ()  [unwired: 1 out]
      n400 = local read "输入值_75"() -> ()  [unwired: 1 out]
      n401 = local read "输入值_76"() -> ()  [unwired: 1 out]
      n402 = local read "输入值_77"() -> ()  [unwired: 1 out]
      n403 = local read "输入值_78"() -> ()  [unwired: 1 out]
      n404 = local read "输入值_79"() -> ()  [unwired: 1 out]
      n405 = local read "输入值_80"() -> ()  [unwired: 1 out]
    }
    frame Enabled {
    }
  }
  n406 = stacked-sequence {
    frame #0 {
      n407 = stacked-sequence {
        frame #0 {
          w4 = T1."Enabled" ("禁用")
          w5 = cluster{u32, u32}[] [{9868950, 9868950}]
          w6 = 0 ("同步_A2")
          w22 = T1."Disabled" ("禁用")
          n408 = property on="测试结论" class="Str"("Text.TextColor"=u32 0) -> ()  [unwired: 2 in, 2 out]
          n409 = local write "测试结论"("") -> ()
          n410 = property on="D_IN_1" class="Tbl (严格)"("DisabledEnum"=w22) -> ()  [unwired: 2 in, 2 out]
          n411 = property on="D_IN_2" class="Tbl (严格)"("DisabledEnum"=w22) -> ()  [unwired: 2 in, 2 out]
          n412 = property on="D_IN_3" class="Tbl (严格)"("DisabledEnum"=w22) -> ()  [unwired: 2 in, 2 out]
          n413 = property on="D_IN_4" class="Tbl (严格)"("DisabledEnum"=w22) -> ()  [unwired: 2 in, 2 out]
          n414 = property on="D_IN_5" class="Tbl (严格)"("DisabledEnum"=w22) -> ()  [unwired: 2 in, 2 out]
          n415 = property on="light_1" class="Bool (严格)"("Colors [4]"=w5) -> ()  [unwired: 2 in, 2 out]
          n416 = property on="light_2" class="Bool (严格)"("Colors [4]"=w5) -> ()  [unwired: 2 in, 2 out]
          n417 = property on="light_3" class="Bool (严格)"("Colors [4]"=w5) -> ()  [unwired: 2 in, 2 out]
          n418 = property on="light_4" class="Bool (严格)"("Colors [4]"=w5) -> ()  [unwired: 2 in, 2 out]
          n419 = property on="light_5" class="Bool (严格)"("Colors [4]"=w5) -> ()  [unwired: 2 in, 2 out]
          n420 = property on="light_6" class="Bool (严格)"("Colors [4]"=w5) -> ()  [unwired: 2 in, 2 out]
          n421 = property on="light_7" class="Bool (严格)"("Colors [4]"=w5) -> ()  [unwired: 2 in, 2 out]
          n422 = property on="light_8" class="Bool (严格)"("Colors [4]"=w5) -> ()  [unwired: 2 in, 2 out]
          n423 = property on="light_9" class="Bool (严格)"("Colors [4]"=w5) -> ()  [unwired: 2 in, 2 out]
          n424 = property on="light_10" class="Bool (严格)"("Colors [4]"=w5) -> ()  [unwired: 2 in, 2 out]
          n425 = property on="light_11" class="Bool (严格)"("Colors [4]"=w5) -> ()  [unwired: 2 in, 2 out]
          n426 = property on="light_12" class="Bool (严格)"("Colors [4]"=w5) -> ()  [unwired: 2 in, 2 out]
          n427 = property on="light_13" class="Bool (严格)"("Colors [4]"=w5) -> ()  [unwired: 2 in, 2 out]
          n428 = property on="light_14" class="Bool (严格)"("Colors [4]"=w5) -> ()  [unwired: 2 in, 2 out]
          n429 = property on="light_15" class="Bool (严格)"("Colors [4]"=w5) -> ()  [unwired: 2 in, 2 out]
          n430 = property on="light_16" class="Bool (严格)"("Colors [4]"=w5) -> ()  [unwired: 2 in, 2 out]
          n431 = property on="light_17" class="Bool (严格)"("Colors [4]"=w5) -> ()  [unwired: 2 in, 2 out]
          n432 = property on="light_18" class="Bool (严格)"("Colors [4]"=w5) -> ()  [unwired: 2 in, 2 out]
          n433 = property on="light_19" class="Bool (严格)"("Colors [4]"=w5) -> ()  [unwired: 2 in, 2 out]
          n434 = property on="light_20" class="Bool (严格)"("Colors [4]"=w5) -> ()  [unwired: 2 in, 2 out]
          n435 = property on="light_21" class="Bool (严格)"("Colors [4]"=w5) -> ()  [unwired: 2 in, 2 out]
          n436 = property on="light_22" class="Bool (严格)"("Colors [4]"=w5) -> ()  [unwired: 2 in, 2 out]
          n437 = property on="light_23" class="Bool (严格)"("Colors [4]"=w5) -> ()  [unwired: 2 in, 2 out]
          n438 = property on="light_24" class="Bool (严格)"("Colors [4]"=w5) -> ()  [unwired: 2 in, 2 out]
          n439 = property on="light_25" class="Bool (严格)"("Colors [4]"=w5) -> ()  [unwired: 2 in, 2 out]
          n440 = property on="light_26" class="Bool (严格)"("Colors [4]"=w5) -> ()  [unwired: 2 in, 2 out]
          n441 = property on="light_27" class="Bool (严格)"("Colors [4]"=w5) -> ()  [unwired: 2 in, 2 out]
          n442 = property on="light_28" class="Bool (严格)"("Colors [4]"=w5) -> ()  [unwired: 2 in, 2 out]
          n443 = property on="light_29" class="Bool (严格)"("Colors [4]"=w5) -> ()  [unwired: 2 in, 2 out]
          n444 = property on="light_30" class="Bool (严格)"("Colors [4]"=w5) -> ()  [unwired: 2 in, 2 out]
          n445 = property on="light_31" class="Bool (严格)"("Colors [4]"=w5) -> ()  [unwired: 2 in, 2 out]
          n446 = property on="light_32" class="Bool (严格)"("Colors [4]"=w5) -> ()  [unwired: 2 in, 2 out]
          n447 = property on="light_33" class="Bool (严格)"("Colors [4]"=w5) -> ()  [unwired: 2 in, 2 out]
          n448 = property on="light_34" class="Bool (严格)"("Colors [4]"=w5) -> ()  [unwired: 2 in, 2 out]
          n449 = property on="light_35" class="Bool (严格)"("Colors [4]"=w5) -> ()  [unwired: 2 in, 2 out]
          n450 = property on="light_36" class="Bool (严格)"("Colors [4]"=w5) -> ()  [unwired: 2 in, 2 out]
          n451 = property on="light_37" class="Bool (严格)"("Colors [4]"=w5) -> ()  [unwired: 2 in, 2 out]
          n452 = property on="light_38" class="Bool (严格)"("Colors [4]"=w5) -> ()  [unwired: 2 in, 2 out]
          n453 = property on="light_39" class="Bool (严格)"("Colors [4]"=w5) -> ()  [unwired: 2 in, 2 out]
          n454 = property on="light_40" class="Bool (严格)"("Colors [4]"=w5) -> ()  [unwired: 2 in, 2 out]
          n455 = property on="light_41" class="Bool (严格)"("Colors [4]"=w5) -> ()  [unwired: 2 in, 2 out]
          n456 = property on="light_42" class="Bool (严格)"("Colors [4]"=w5) -> ()  [unwired: 2 in, 2 out]
          n457 = property on="light_43" class="Bool (严格)"("Colors [4]"=w5) -> ()  [unwired: 2 in, 2 out]
          n458 = property on="light_44" class="Bool (严格)"("Colors [4]"=w5) -> ()  [unwired: 2 in, 2 out]
          n459 = property on="light_45" class="Bool (严格)"("Colors [4]"=w5) -> ()  [unwired: 2 in, 2 out]
          n460 = property on="light_46" class="Bool (严格)"("Colors [4]"=w5) -> ()  [unwired: 2 in, 2 out]
          n461 = property on="light_47" class="Bool (严格)"("Colors [4]"=w5) -> ()  [unwired: 2 in, 2 out]
          n462 = property on="light_48" class="Bool (严格)"("Colors [4]"=w5) -> ()  [unwired: 2 in, 2 out]
          n463 = property on="light_49" class="Bool (严格)"("Colors [4]"=w5) -> ()  [unwired: 2 in, 2 out]
          n464 = property on="light_50" class="Bool (严格)"("Colors [4]"=w5) -> ()  [unwired: 2 in, 2 out]
          n465 = property on="light_51" class="Bool (严格)"("Colors [4]"=w5) -> ()  [unwired: 2 in, 2 out]
          n466 = property on="light_52" class="Bool (严格)"("Colors [4]"=w5) -> ()  [unwired: 2 in, 2 out]
          n467 = property on="light_53" class="Bool (严格)"("Colors [4]"=w5) -> ()  [unwired: 2 in, 2 out]
          n468 = property on="light_54" class="Bool (严格)"("Colors [4]"=w5) -> ()  [unwired: 2 in, 2 out]
          n469 = property on="light_55" class="Bool (严格)"("Colors [4]"=w5) -> ()  [unwired: 2 in, 2 out]
          n470 = property on="light_56" class="Bool (严格)"("Colors [4]"=w5) -> ()  [unwired: 2 in, 2 out]
          n471 = property on="light_57" class="Bool (严格)"("Colors [4]"=w5) -> ()  [unwired: 2 in, 2 out]
